vi "Number To Decimal String Conversion part 10.vi"() -> ()   [LabVIEW 2020]
panel:
  out "concatenated string":string
  in  "number":i32
  in  "String":string
  # "Number To Decimal String Conversion"
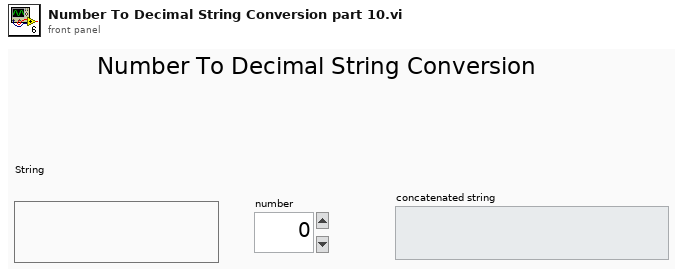
[diagram p1: front panel]
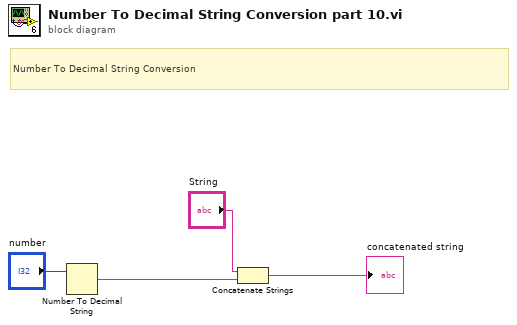
[diagram p0: block diagram]
diagram:
  # "Number To Decimal String Conversion"
  n1 = Number To Decimal String(number="number") -> (decimal integer string=w3:string)  [unwired: 1 in]
  n2 = Concatenate Strings "Concatenate Strings"("String", w3) -> (→"concatenated string":string)
